vi "DFD M-Band Filter Bank Reconstruction.vi"   [LabVIEW 2017, in "NI_DigFilter_FilterBank.lvlib"]
doc: "Reconstructs a signal from M-band subband signals continuously with a cosine-modulated filter bank."
uses:
  <vilib>/addons/Digital Filter Design/NI_DigFilter_FilterBank.lvlib
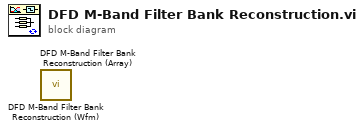
[diagram p0: block diagram]
diagram:
  n1 = call <vilib>:"DFD M-Band Filter Bank Reconstruction (Wfm).vi"() -> ()  [unwired: 10 in, 2 out]
  n2 = call <vilib>:"DFD M-Band Filter Bank Reconstruction (Array).vi"() -> ()  [unwired: 10 in, 2 out]
